vi "UpdateMeasurementValues.vi"(8 "Error in":errorcluster, 10 "DaqMeasurement":refnum<k24>, 11 "DevicesAndSignals":T1) -> (0 "Error out":errorcluster, 2 "DaqMeasurement":refnum<k24>, 3 "DevicesAndSignals":T1)   [LabVIEW 2016]
doc: "Updates the signals measurement values. Call this function periodically during a measurement.\n\nThis function updates all measurement values of all signals that take part in measuring. \nIn case of a synchronized start of data acquisition, it asserts that each signal with same sample rate (distributed to various devices) gets the same number of new measuring values. E.g. signal_A on device 1 with sample rate 20Hz gets the same number of new measurement values as signal_B on device 2 with sample rate 20 Hz! \nOtherwise (if StartDaq started an unsynchronized measurement, the signals get all measurement values that are accumulated since the last call of this function. \nThis function also asserts, that there is enough allocated memory for the measurement values of each signal."
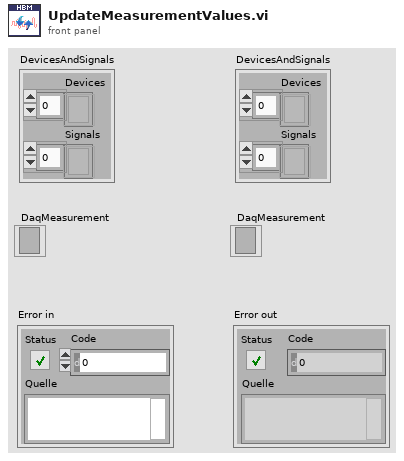
[diagram p1: front panel]
types:
  T1 = cluster{"Devices":refnum<k24>[], "Signals":refnum<k24>[]}
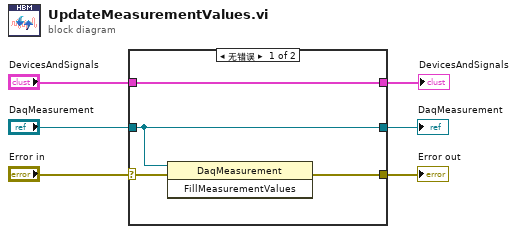
[diagram p0: block diagram]
diagram:
  n1 = case shown="无错误" "Error in" {
    selector: "Error in" -> [w10 w13]
    tunnel: "DaqMeasurement" -> [w9 w11]
    tunnel: "DevicesAndSignals" -> [w8 w12]
    tunnel: [w7 w13] -> w3
    tunnel: [w8 w12] -> w2
    tunnel: [w9 w11] -> w1
    frame No Error {
      n2 = invoke on="Methodenknoten" class="DaqMeasurement" method="FillMeasurementValues"(reference=w9, error in=w10) -> (error out=w7:errorcluster)  [unwired: 1 in, 2 out]
    }
    frame Error {
    }
  }
  "Error out" <- w3
  "DevicesAndSignals" <- w2
  "DaqMeasurement" <- w1
